vi "MPXsetFrequence.vi"(2 "Refresh":bool, 3 "Frequence [Hz]":i32=10, 4 "Comport in":refnum<visa-resource-name>="COM5") -> (0 "read buffer":string="boff\r\nSignal off\r\n\r\nWavetype: Sine\r\nFrequence: 0125 Hz\r\nAmplitude: 198,0 V\r\nSignal off\r\n\r\nempc>:\n", 1 "Comport out":refnum<visa-resource-name>="COM5")   [LabVIEW 2015]
uses:
  Instance           1 24Saved   MPX setFrequence .vi
panel:
  out "Frequence bkp":i32=10
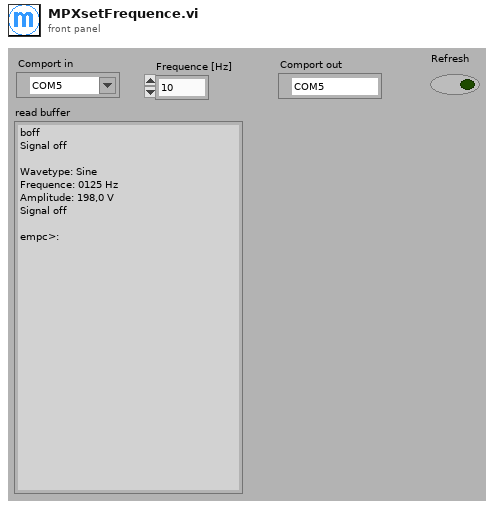
[diagram p1: front panel]
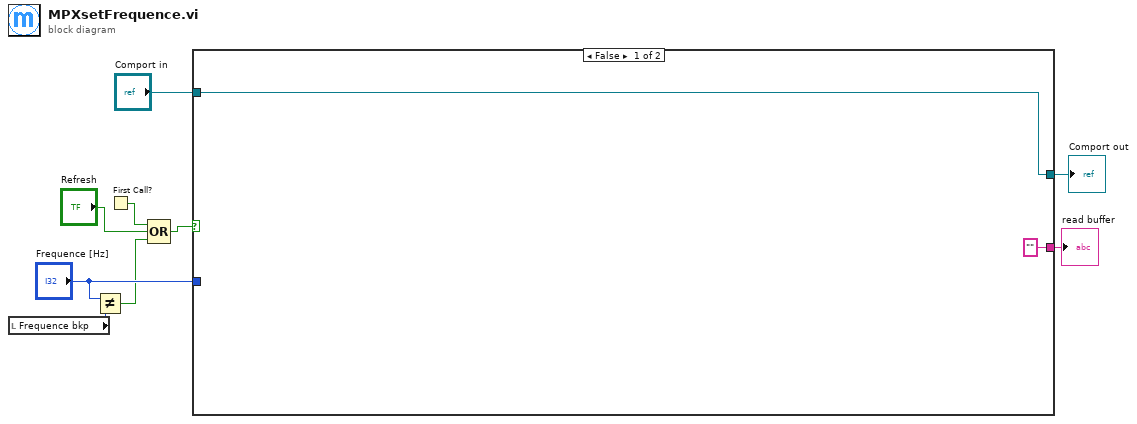
[diagram p0: block diagram]
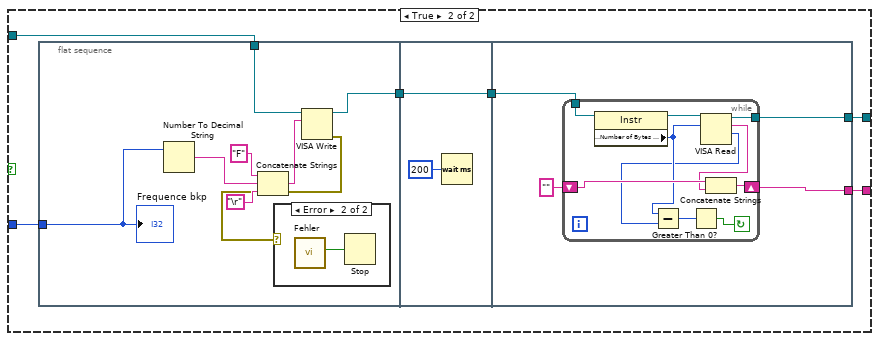
[diagram p2: hidden frame]
diagram:
  n1 = local read "Frequence bkp"() -> (w3:i32)
  n2 = Not Equal?(x="Frequence [Hz]", y=w3) -> (x != y?=w2:bool)
  n3 = First Call?() -> (First Call?: T/F=w5:bool)
  n4 = Compound Arithmetic op=OR(w5, "Refresh", w2) -> (w7:bool)
  n5 = case shown="False" w7 {
    tunnel: "Comport in" -> [w11 w15]
    tunnel: [w11 w14] -> w8
    tunnel: "Frequence [Hz]" -> [_ w13]
    tunnel: ["" w12] -> w1
    frame False {
    }
    frame True {
      n6 = flat-sequence {
        tunnel: w15 -> [w21]
        tunnel: [w18] -> w17
        tunnel: w13 -> [w20]
        tunnel: w17 -> [w27]
        tunnel: [w27] -> w16
        tunnel: w16 -> [w32]
        tunnel: [w30] -> w14
        tunnel: [w29] -> w12
        frame #0 {
          n7 = Number To Decimal String(number=w20) -> (decimal integer string=w22:string)  [unwired: 1 in]
          n8 = Concatenate Strings("F", w22, "\r") -> (w25:string)
          n9 = VISA Write(VISA resource name=w21, write buffer=w25) -> (VISA resource name out=w18:refnum<visa-resource-name>, error out=w19:errorcluster)  [unwired: 1 in, 1 out]
          n10 = case shown="Error" w19 {
            frame No Error {
            }
            frame Error {
              n11 = call "Fehler"() -> ("OK"=w26:bool)  [unwired: 10 in, 1 out]
              n12 = Stop(stop? (T)=w26) -> ()
            }
          }
          "Frequence bkp" <- w20
        }
        frame #1 {
          n13 = Wait (ms)(milliseconds to wait=u32 200) -> ()  [unwired: 1 out]
        }
        frame #2 {
          n14 = while {
            shift-right: [w40] -> w29
            shift-left: "" -> [w41]
            tunnel: w32 -> [w34]
            tunnel: [w33] -> w30
            stop <- w35 continue-if-true
            n15 = property class="Instr"(reference=w34) -> (reference out=w42:refnum<visa-resource-name>, "Serial Settings:Number of Bytes at Serial Port"=w37:u32)  [unwired: 1 in, 1 out]
            n16 = VISA Read(VISA resource name=w42, byte count=w37) -> (VISA resource name out=w33:refnum<visa-resource-name>, read buffer=w39:string, return count=w36:u32)  [unwired: 1 in, 1 out]
            n17 = Subtract(x=w37, y=w36) -> (x-y=w38:u32)
            n18 = Greater Than 0?(x=w38) -> (x > 0?=w35:bool)
            n19 = Concatenate Strings(w41, w39) -> (w40:string)
          }
        }
      }
    }
  }
  "Comport out" <- w8
  "read buffer" <- w1
